vi "Plot de gráficos.vi"() -> ()   [LabVIEW 2014]
panel:
  out "XY Graph":cluster{"X":dbl[], "Y":dbl[]}[](graph)
  out "Função - Cos":cluster{"Y":dbl[], "Y":dbl[]}[](graph)
  out "Função - 2^x":cluster{"Y":dbl[], "Y":dbl[]}[](graph)
  out "Função - X²":cluster{"Y":dbl[], "Y":dbl[]}[](graph)
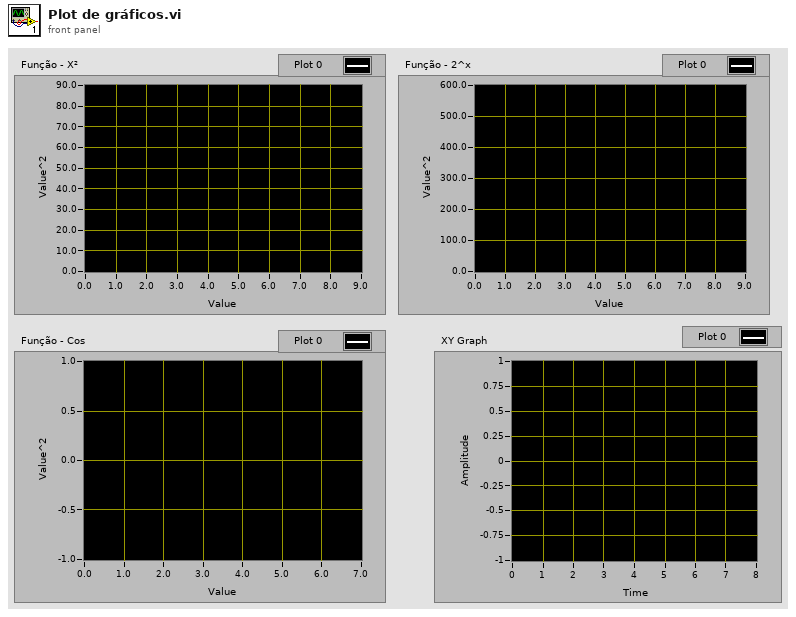
[diagram p1: front panel]
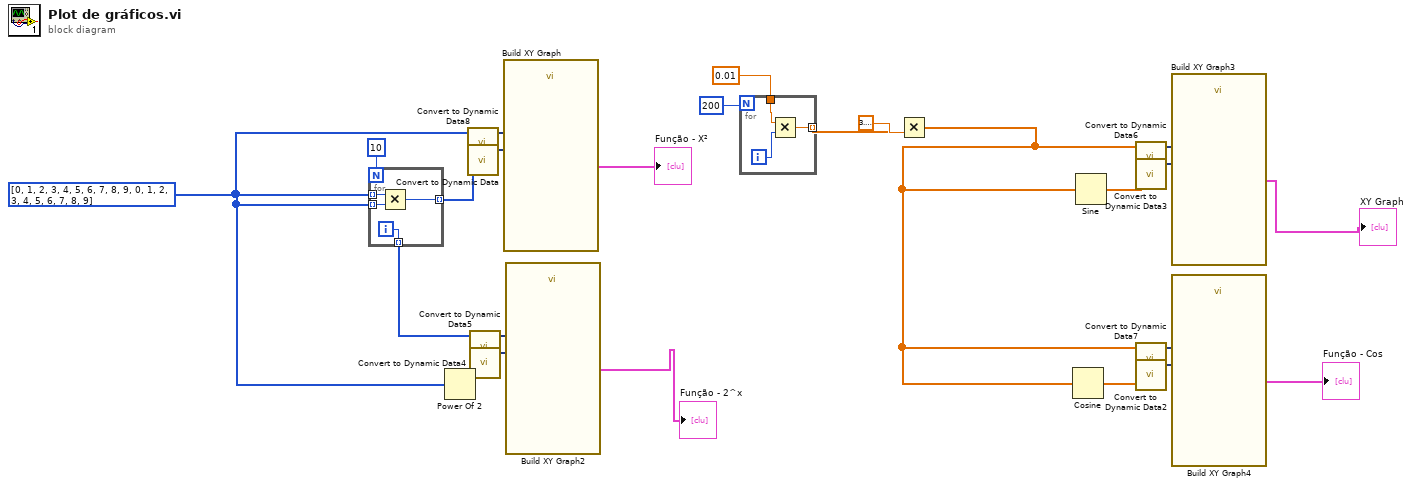
[diagram p0: block diagram]
diagram:
  w2 = i32[] [0, 1, 2, 3, 4, 5, 6, 7, 8, 9, 0, 1, 2, 3, 4, 5, 6, 7, 8, 9]
  n1 = for {
    N: 10 -> [_]
    tunnel: [w28] -> w18 mode=indexing
    tunnel: w2 -> [w27] mode=indexing
    tunnel: w2 -> [w26] mode=indexing
    tunnel: [w25] -> w1 mode=indexing
    i -> [w25]
    n2 = Multiply(x=w27, y=w26) -> (x*y=w28:i32)
  }
  n3 = Power Of 2(x=w2) -> (2^x=w19:dbl[])
  n4 = call "Convert to Dynamic Data8"("Array"=w2) -> ("Dynamic Data Type"=w10:dynamicdata)  [unwired: 3 in]
  n5 = call "Convert to Dynamic Data"("Array"=w18) -> ("Dynamic Data Type"=w17:dynamicdata)  [unwired: 3 in]
  n6 = call "Convert to Dynamic Data5"("Array"=w1) -> ("Dynamic Data Type"=w13:dynamicdata)  [unwired: 3 in]
  n7 = call "Convert to Dynamic Data4"("Array"=w19) -> ("Dynamic Data Type"=w14:dynamicdata)  [unwired: 3 in]
  n8 = call "Build XY Graph"("Y Input"=w17, "X Input"=w10) -> ("XY Graph"=→"Função - X²":cluster{"X":dbl[], "Y":dbl[]}[])  [unwired: 8 in, 1 out]
  n9 = call "Build XY Graph2"("Y Input"=w14, "X Input"=w13) -> ("XY Graph"=→"Função - 2^x":cluster{"X":dbl[], "Y":dbl[]}[])  [unwired: 8 in, 1 out]
  n10 = for {
    N: 200 -> [_]
    tunnel: [w30] -> w4 mode=indexing
    tunnel: 0.01 -> [w29]
    i -> [w31]
    n11 = Multiply(x=w29, y=w31) -> (x*y=w30:dbl)
  }
  n12 = Multiply(x=w4, y=3.141592653589793) -> (x*y=w6:dbl[])
  n13 = Cosine(x=w6) -> (cos(x)=w21:dbl[])
  n14 = Sine(x=w6) -> (sin(x)=w20:dbl[])
  n15 = call "Convert to Dynamic Data6"("Array"=w6) -> ("Dynamic Data Type"=w12:dynamicdata)  [unwired: 3 in]
  n16 = call "Convert to Dynamic Data3"("Array"=w20) -> ("Dynamic Data Type"=w15:dynamicdata)  [unwired: 3 in]
  n17 = call "Convert to Dynamic Data7"("Array"=w6) -> ("Dynamic Data Type"=w11:dynamicdata)  [unwired: 3 in]
  n18 = call "Convert to Dynamic Data2"("Array"=w21) -> ("Dynamic Data Type"=w16:dynamicdata)  [unwired: 3 in]
  n19 = call "Build XY Graph3"("Y Input"=w15, "X Input"=w12) -> ("XY Graph"=→"XY Graph":cluster{"X":dbl[], "Y":dbl[]}[])  [unwired: 8 in, 1 out]
  n20 = call "Build XY Graph4"("Y Input"=w16, "X Input"=w11) -> ("XY Graph"=→"Função - Cos":cluster{"X":dbl[], "Y":dbl[]}[])  [unwired: 8 in, 1 out]
